vi "get Command Data Element.vi"(8 "error in (no error)":errorcluster, 11 "REx - CMD_TEMPLATE in":refnum<class "Alpha Cmd.lvclass">) -> (0 "error out":errorcluster, 2 "Command Data Element":T1, 3 "REx - CMD_TEMPLATE out":refnum<class "Alpha Cmd.lvclass">)   [LabVIEW 2012, in "Alpha Cmd.lvclass"]
uses:
  Alpha Cmd.lvclass
  STYP - Command Data Element.ctl
  Alpha Cmd.lvclass/Alpha Cmd.ctl
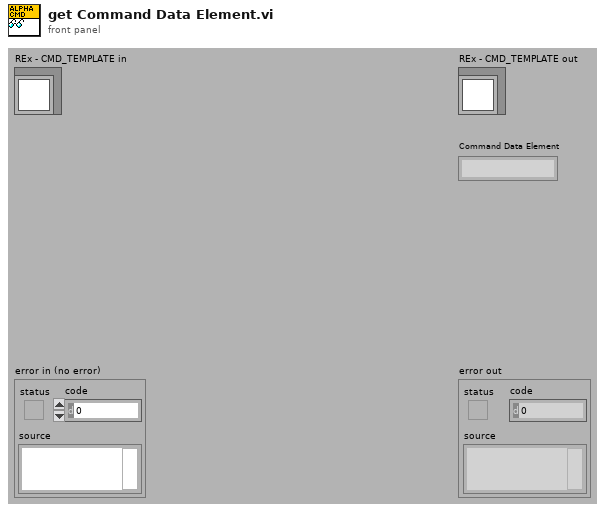
[diagram p1: front panel]
types:
  T1 = typedef "Alpha Cmd.lvclass/STYP - Command Data Element.ctl" = string
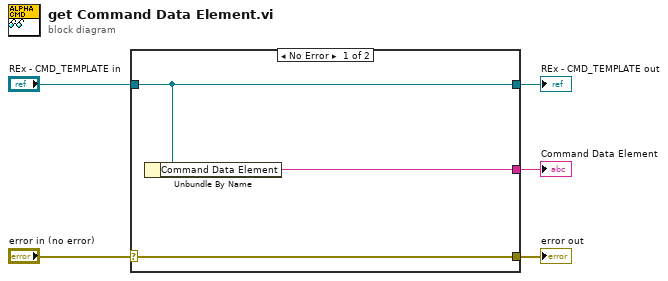
[diagram p0: block diagram]
diagram:
  n1 = case shown="No Error" "error in (no error)" {
    selector: "error in (no error)" -> [w8 w9]
    tunnel: [w8 w9] -> w4
    tunnel: [w7 w10] -> w2
    tunnel: "REx - CMD_TEMPLATE in" -> [w7 w10]
    tunnel: [w6 _] -> w1
    frame No Error {
      n2 = Unbundle By Name(w7) -> ("Command Data Element"=w6:T1)
    }
    frame Error {
    }
  }
  "error out" <- w4
  "REx - CMD_TEMPLATE out" <- w2
  "Command Data Element" <- w1
